vi "ManMarkZagueiro.vi"(8 "Our Robot":T1={"id"=0, "function"=enum."Attacker", "x"=0.0, "y"=0.0, "orientation"=0.0, "v_tangent"=0.0, "v_normal"=0.0, "v_ang"=0.0, "kick_x"=0.0, "kick_z"=0.0, "dribble"=FALSE, "Timestamp"=timestamp(0 s since 1904-01-01), "estimatives"={"est_v_tangent"=0.0, "est_v_normal"=0.0, "est_vx"=0.0, "est_vy"=0.0, "Pos Robot Est"=[]}, "dest_x_kick"=0.0, "dest_y_kick"=0.0, "Gap Coord"=[], "States"=enum."GoToTangent", "Path "=[], "Path  Smooth"=[], "Dest"=[]}, 10 "IA Input":T6={"our_robots"=[], "enemy_robots"=[], "balls"=[], "geometry"={"line_width"=0, "field_length"=0, "field_width"=0, "boundary_width"=0, "referee_width"=0, "goal_width"=0, "goal_depth"=0, "goal_wall_width"=0, "center_circle_radius"=0, "defense_radius"=0, "defense_stretch"=0, "free_kick_from_defense_dist"=0, "penalty_spot_from_field_line_dist"=0, "penalty_line_from_spot_dist"=0}, "IA Judge"={"stage"="", "command"="", "our_goalie_id"=0.0, "enemy_goalie_id"=0.0, "command enum"=enum."Halt", "Time"=enum."Azul"}, "Received Timestamp"=timestamp(0 s since 1904-01-01), "Events"={"Touch"=FALSE, "Ball out"=FALSE, "id touch"=0.0, "Ball out of \nVision"=FALSE, "Ball inside \nGoalie area"=FALSE, "Robot not responding"=FALSE, "Robots responding status"=[1.0, 1.0, 1.0, 1.0, 1.0, 1.0], "Enemy Ball \nPossession"=FALSE, "Pass State"=FALSE, "id end of pass"=0.0, "Kick"=FALSE, "Id ini Possession"=0.0, "Ball Possesion"=FALSE, "Id Possesion"=0.0}}) -> (2 "Robot out":T1={"id"=0, "function"=enum."Attacker", "x"=0.0, "y"=0.0, "orientation"=0.0, "v_tangent"=0.0, "v_normal"=0.0, "v_ang"=0.0, "kick_x"=0.0, "kick_z"=0.0, "dribble"=FALSE, "Timestamp"=timestamp(0 s since 1904-01-01), "estimatives"={"est_v_tangent"=0.0, "est_v_normal"=0.0, "est_vx"=0.0, "est_vy"=0.0, "Pos Robot Est"=[]}, "dest_x_kick"=0.0, "dest_y_kick"=0.0, "Gap Coord"=[], "States"=enum."GoToTangent", "Path "=[], "Path  Smooth"=[], "Dest"=[]})   [LabVIEW 2017]
uses:
  Core/AI Input.ctl
  Core/AI Robot.ctl
  Functions Enum.ctl
  AttackerStates.ctl
  Path Planning/RRT/PathDests.ctl
  Path Planning/RRT/PathDest.ctl
  Core/AI Ball.ctl
  Core/Field Size.ctl
  Core/AI Judge.ctl
  Command Enum.ctl
  Util/Events/Events.ctl
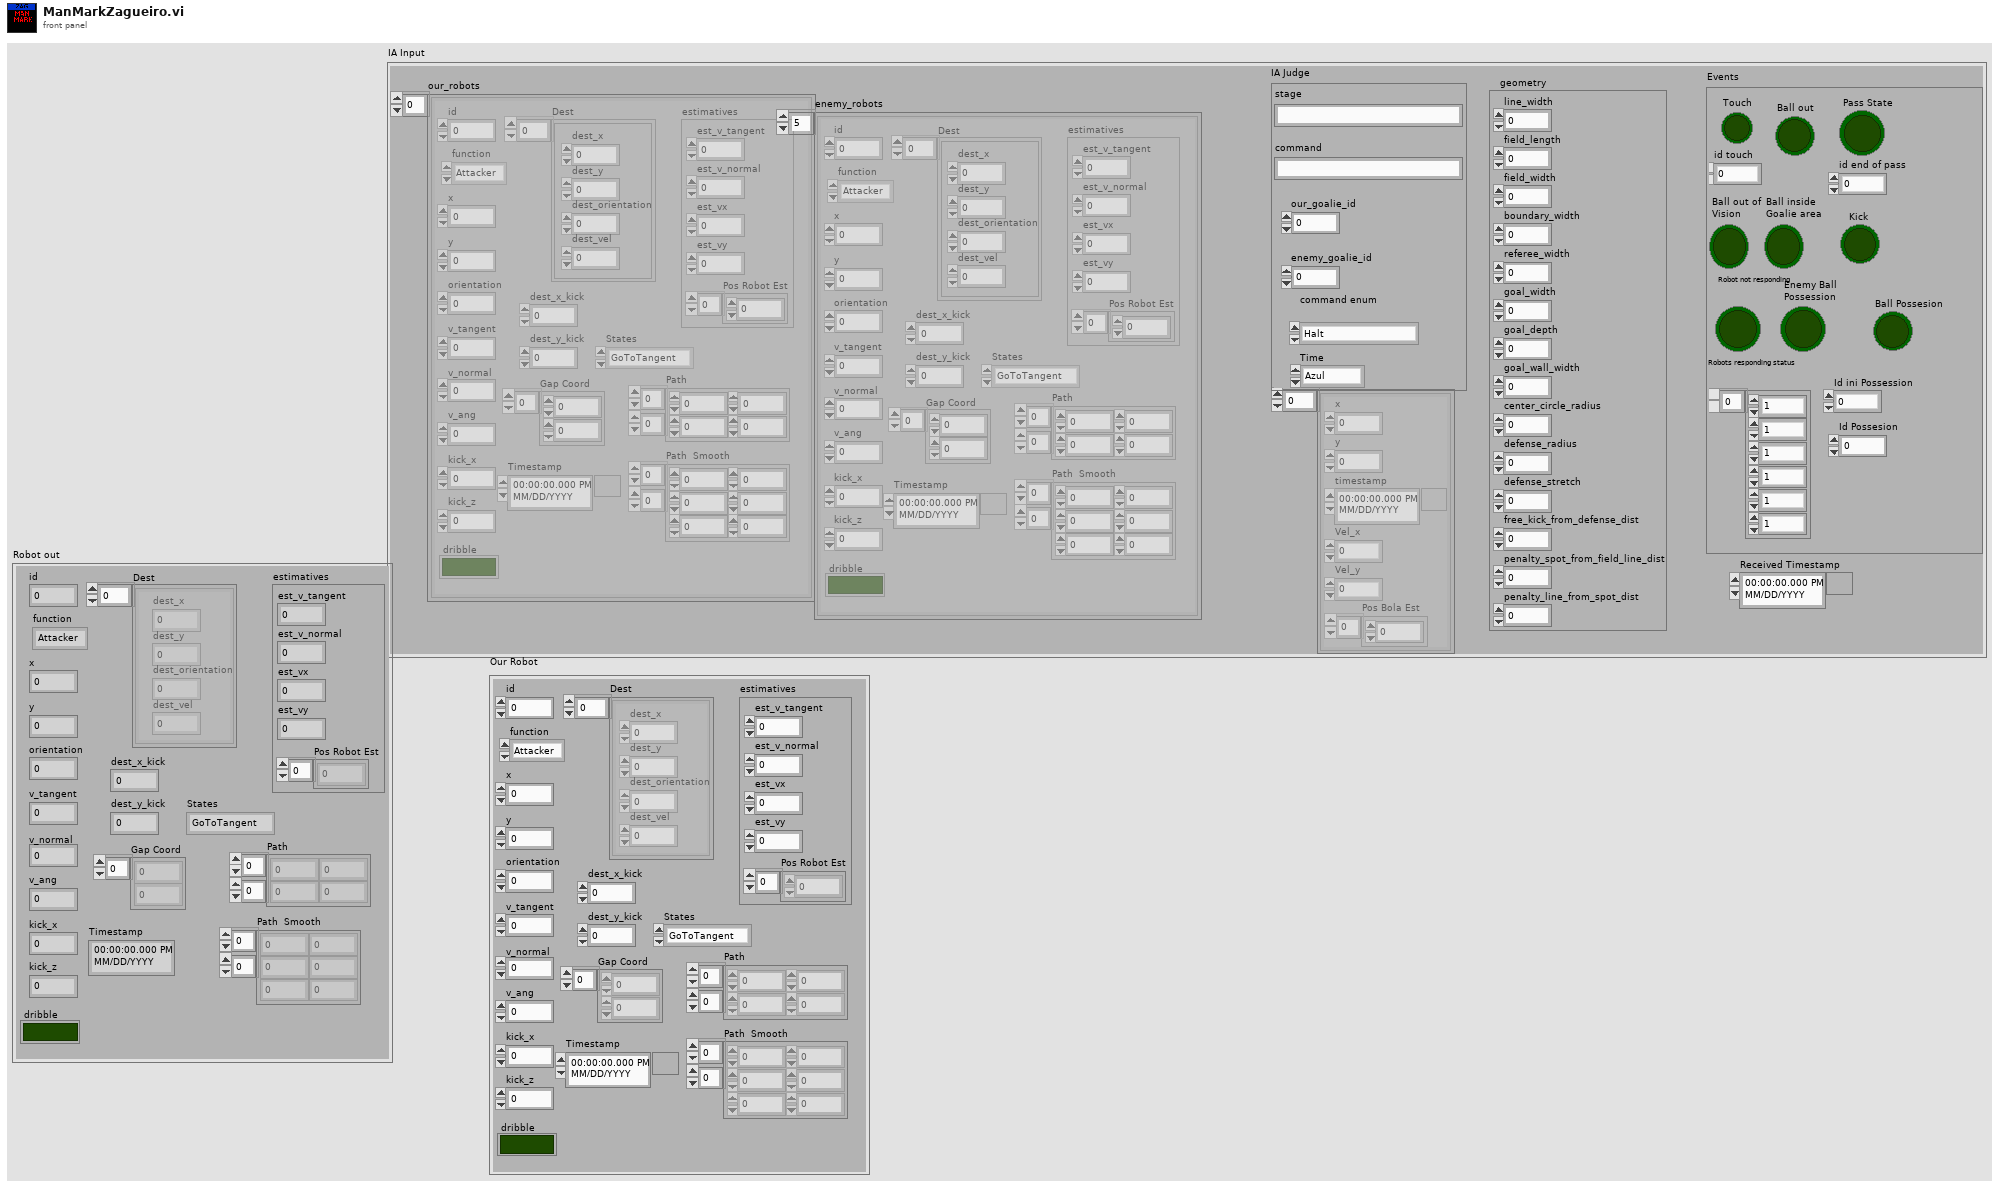
[diagram p1: front panel]
types:
  T1 = typedef "AI Robot.ctl" = cluster{"id":u32, "function":T2, "x":dbl, "y":dbl, "orientation":dbl, "v_tangent":dbl, "v_normal":dbl, "v_ang":dbl, "kick_x":dbl, "kick_z":dbl, "dribble":bool, "Timestamp":timestamp, "estimatives":cluster{"est_v_tangent":dbl, "est_v_normal":dbl, "est_vx":dbl, "est_vy":dbl, "Pos Robot Est":dbl[]}, "dest_x_kick":dbl, "dest_y_kick":dbl, "Gap Coord":dbl[], "States":T3, "Path ":dbl[][], "Path  Smooth":dbl[][], "Dest":T4}
  T2 = typedef "Functions Enum.ctl" = enum16{"Attacker", "Goalie", "Defender", "Striker", "Goto 0", "Dummy", "Kicker", "ZigZag"}
  T3 = typedef "AttackerStates.ctl" = enum16{"Pass", "GoToTangent", "BallGetting", "GoToKick", ""}
  T4 = typedef "PathDests.ctl" = T5[]
  T5 = typedef "PathDest.ctl" = cluster{"dest_x":dbl, "dest_y":dbl, "dest_orientation":dbl, "dest_vel":dbl}
  T6 = typedef "AI Input.ctl" = cluster{"our_robots":T1[], "enemy_robots":T1[], "balls":T7[], "geometry":T8, "IA Judge":T9, "Received Timestamp":timestamp, "Events":T11}
  T7 = typedef "AI Ball.ctl" = cluster{"x":dbl, "y":dbl, "timestamp":timestamp, "Vel_x":dbl, "Vel_y":dbl, "Pos Bola Est":dbl[]}
  T8 = typedef "Field Size.ctl" = cluster{"line_width":u32, "field_length":u32, "field_width":u32, "boundary_width":u32, "referee_width":u32, "goal_width":u32, "goal_depth":u32, "goal_wall_width":u32, "center_circle_radius":u32, "defense_radius":u32, "defense_stretch":u32, "free_kick_from_defense_dist":u32, "penalty_spot_from_field_line_dist":u32, "penalty_line_from_spot_dist":u32}
  T9 = typedef "AI Judge.ctl" = cluster{"stage":string, "command":string, "our_goalie_id":dbl, "enemy_goalie_id":dbl, "command enum":T10, "Time":enum16{"Azul", "Amarelo"}}
  T10 = typedef "Command Enum.ctl" = enum16{"Halt", "Stop", "Force Start", "PKA Normal Start", "Prepare Kickoff Ally", "PKE Normal Start", "Prepare Kickoff Enemy", "Prepare Penalty Ally", "PPA Normal Start", "Prepare Penalty Enemy", "PPE Normal Start", "Direct Free Enemy", "Direct Free Ally", "Indirect Free Enemy", "Indirect Free Ally", "Timeout Enemy", "Timeout Ally", "Goal Enemy", "Goal Ally", "Ball Placement Enemy", "Ball Placement Ally", "Normal Half Time", "Extra Time Break", "Extra Half Time", "None", "Post Game"}
  T11 = typedef "Events.ctl" = cluster{"Touch":bool, "Ball out":bool, "id touch":dbl, "Ball out of \nVision":bool, "Ball inside \nGoalie area":bool, "Robot not responding":bool, "Robots responding status":dbl[], "Enemy Ball \nPossession":bool, "Pass State":bool, "id end of pass":dbl, "Kick":bool, "Id ini Possession":dbl, "Ball Possesion":bool, "Id Possesion":dbl}
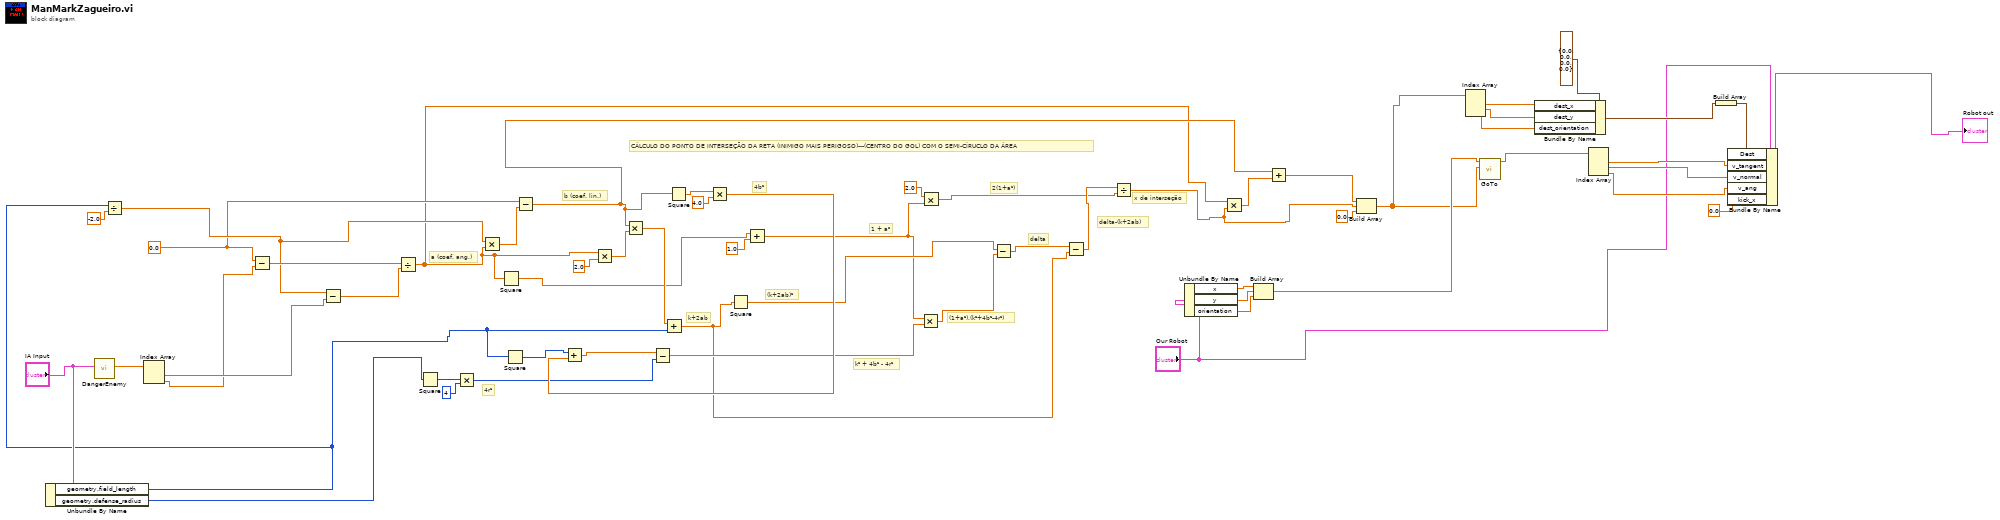
[diagram p0: block diagram]
diagram:
  w30 = 0.0
  # "x de interseção"
  # "CÁLCULO DO PONTO DE INTERSEÇÃO DA RETA (INIMIGO MAIS PERIGOSO)---(CENTRO DO GOL) COM O SEMI-CÍRUCLO DA ÁREA"
  # "delta-(k+2ab)"
  # "2(1+a²)"
  # "delta"
  # "(1+a²).(k²+4b²-4r²)"
  # "(k+2ab)²"
  # "k+2ab"
  # "k² + 4b² - 4r²"
  # "1 + a²"
  # "4r²"
  # "4b²"
  # "b (coef. lin.)"
  # "a (coef. ang.)"
  n1 = Unbundle By Name("IA Input") -> ("geometry.field_length"=w4:u32, "geometry.defense_radius"=w3:u32)
  n2 = call "DangerEnemy.vi"("IA Input"="IA Input") -> ("Pos do inimigo\nperigoso"=w29:dbl[])  [unwired: 7 in, 3 out]
  n3 = Divide(x=w4, y=-2.0) -> (x/y=w31:dbl)
  n4 = Index Array(array=w29) -> (element #1=w28:dbl, element #2=w27:dbl)  [unwired: 2 in]
  n5 = Subtract(x=w30, y=w27) -> (x-y=w58:dbl)
  n6 = Subtract(x=w31, y=w28) -> (x-y=w57:dbl)
  n7 = Divide(x=w58, y=w57) -> (x/y=w26:dbl)
  n8 = Square(x=w3) -> (x^2=w46:u32)
  n9 = Multiply(x=w46, y=u32 4) -> (x*y=w33:u32)
  n10 = Multiply(x=w31, y=w26) -> (x*y=w56:dbl)
  n11 = Square(x=w26) -> (x^2=w51:dbl)
  n12 = Square(x=w4) -> (x^2=w50:u32)
  n13 = Subtract(x=w30, y=w56) -> (x-y=w34:dbl)
  n14 = Multiply(x=w26, y=2.0 ("x")) -> (x*y=w54:dbl)
  n15 = Multiply(x=w34, y=w54) -> (x*y=w53:dbl)
  n16 = Add(x=w53, y=w4) -> (x+y=w39:dbl)
  n17 = Square(x=w34) -> (x^2=w49:dbl)
  n18 = Multiply(x=w49, y=4.0 ("x")) -> (x*y=w47:dbl)
  n19 = Add(x=w50, y=w47) -> (x+y=w44:dbl)
  n20 = Subtract(x=w44, y=w33) -> (x-y=w43:dbl)
  n21 = Square(x=w39) -> (x^2=w42:dbl)
  n22 = Add(x=w51, y=1.0) -> (x+y=w38:dbl)
  n23 = Multiply(x=w38, y=w43) -> (x*y=w41:dbl)
  n24 = Multiply(x=2.0 ("y"), y=w38) -> (x*y=w35:dbl)
  n25 = Subtract(x=w42, y=w41) -> (x-y=w40:dbl)
  n26 = Subtract(x=w40, y=w39) -> (x-y=w36:dbl)
  n27 = Divide(x=w36, y=w35) -> (x/y=w1:dbl)
  n28 = Unbundle By Name("Our Robot") -> ("x"=w22:dbl, "y"=w21:dbl, "orientation"=w20:dbl)
  n29 = Multiply(x=w26, y=w1) -> (x*y=w25:dbl)
  n30 = Build Array(w22, w21, w20) -> (w19:dbl[])
  n31 = Add(x=w34, y=w25) -> (x+y=w24:dbl)
  n32 = Build Array(w24, w1, 0.0 ("element")) -> (w17:dbl[])
  n33 = Index Array(array=w17) -> (element #1=w15:dbl, element #2=w14:dbl, element #3=w13:dbl)  [unwired: 3 in]
  n34 = call "GoTo.vi"("Target"=w17, "Position"=w19) -> ("Output\nVelocity"=w18:dbl[])  [unwired: 8 in, 1 out]
  n35 = Bundle By Name(cluster=T5 {"dest_x"=0.0, "dest_y"=0.0, "dest_orientation"=0.0, "dest_vel"=0.0} ("element"), "dest_x"=w15, "dest_y"=w14, "dest_orientation"=w13) -> (w11:T5)
  n36 = Index Array(array=w18) -> (element #1=w10:dbl, element #2=w9:dbl, element #3=w8:dbl)  [unwired: 3 in]
  n37 = Build Array(w11) -> (w12:T5[])
  n38 = Bundle By Name(cluster="Our Robot", "Dest"=w12, "v_tangent"=w10, "v_normal"=w9, "v_ang"=w8, "kick_x"=0.0) -> (→"Robot out":T1)
